vi "testErrorMessageContainsCustomMessage.vi"(9 "message":string, 10 "expected":string="My error message!") -> (0 "error out":errorcluster)   [LabVIEW 2017, in "Transparent Assertions.Tests.lvlib" / "ExpectationFailedError.lvlib"]
uses:
  ExpectationFailedError.lvlib
  src/Transparent Assertions/Transparent Assertions.lvlib
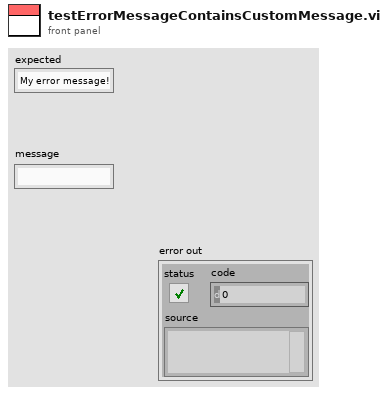
[diagram p1: front panel]
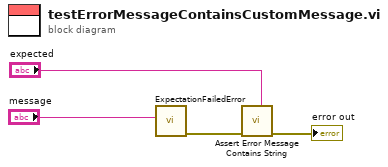
[diagram p0: block diagram]
diagram:
  n1 = call "ExpectationFailedError.vi"("Message"="message") -> ("error out"=w1:errorcluster)  [unwired: 10 in]
  n2 = call "Assert Error Message Contains String.vi"("Expected"="expected", "error in (no error)"=w1) -> ("error out"=→"error out":errorcluster)  [unwired: 9 in]
